vi "Chart & build.vi"() -> ()   [LabVIEW 2012]
panel:
  out "Waveform Chart 2":dbl[](graph)
  out "Array 4":dbl[](array[numeric]) format="%.2f"
  out "Array 3":dbl[](array[numeric]) format="%.2f"
  out "Array 2":dbl[][](array[numeric]) format="%.2f"
  out "Array":dbl[](array[numeric]) format="%.2f"
  out "Waveform Chart":dbl[][](graph)
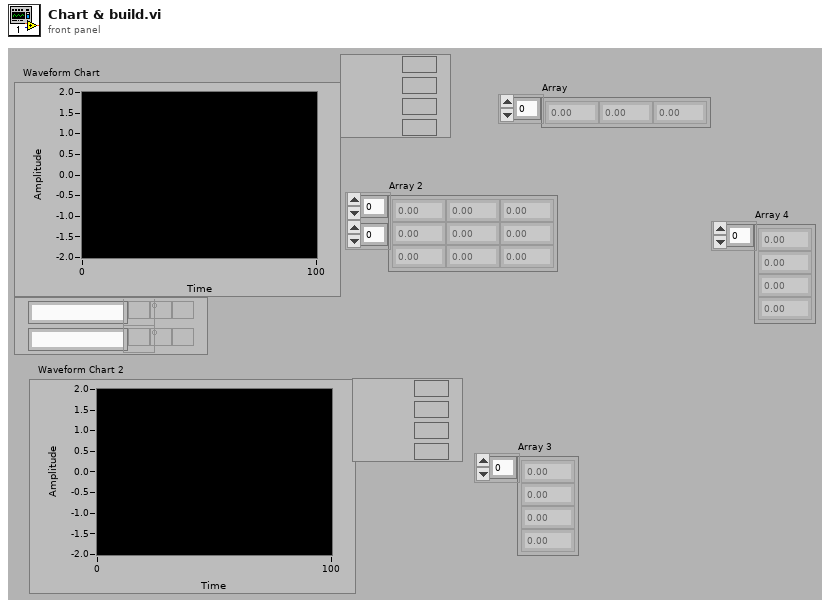
[diagram p1: front panel]
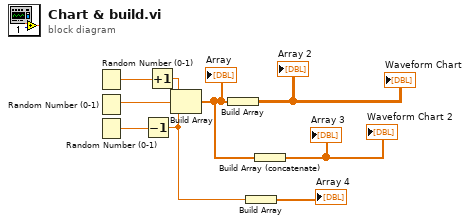
[diagram p0: block diagram]
diagram:
  n1 = Random Number (0-1)() -> (number: 0 to 1=w9:dbl)
  n2 = Random Number (0-1)() -> (number: 0 to 1=w7:dbl)
  n3 = Random Number (0-1)() -> (number: 0 to 1=w3:dbl)
  n4 = Decrement(x=w3) -> (x-1=w2:dbl)
  n5 = Increment(x=w9) -> (x+1=w8:dbl)
  n6 = Build Array(w8, w7, w2) -> (w6:dbl[])
  "Array" <- w6
  n7 = Build Array(w6) -> (→"Waveform Chart" →"Array 2":dbl[][])
  n8 = Build Array(w2) -> (→"Array 4":dbl[])
  n9 = Build Array (concatenate)(w6) -> (→"Array 3" →"Waveform Chart 2":dbl[])
